vi "tau0.vi"(8 "D":sgl, 11 "Xm":sgl) -> (2 "tau0":sgl)   [LabVIEW 2019]
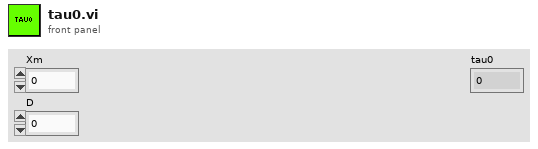
[diagram p1: front panel]
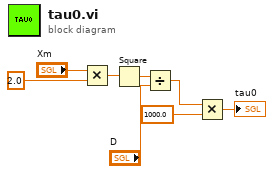
[diagram p0: block diagram]
diagram:
  n1 = Multiply(x="Xm", y=sgl 2.0) -> (x*y=w6:sgl)
  n2 = Square(x=w6) -> (x^2=w5:sgl)
  n3 = Divide(x=w5, y="D") -> (x/y=w3:sgl)
  n4 = Multiply(x=w3, y=sgl 1000.0) -> (x*y=→"tau0":sgl)
